vi "Close CAN Communication queues.vi"(8 "error in":errorcluster, 11 "CAN Session In":T1) -> (0 "error out":errorcluster)   [LabVIEW 2016]
uses:
  Typedefs/CAN Refnum.ctl
  Typedefs/CAN Session Pointer.ctl
  Typedefs/CAN Communication References.ctl
  Typedefs/kill process notifier array.ctl
  Typedefs/Write Queue.ctl
  Typedefs/FPGA CAN Frame Cluster.ctl
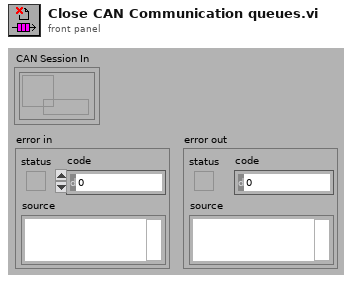
[diagram p1: front panel]
types:
  T1 = typedef "CAN Refnum.ctl" = refnum<k1>
  T2 = typedef "kill process notifier array.ctl" = refnum<notifier>[]
  T3 = typedef "Write Queue.ctl" = refnum<queue>
  T4 = typedef "CAN Session Pointer.ctl" = refnum<queue>
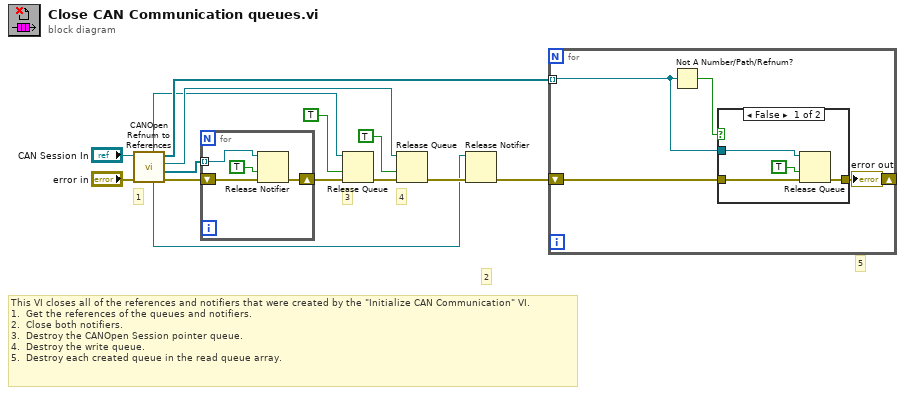
[diagram p0: block diagram]
diagram:
  # "This VI closes all of the references and notifiers that were created by the \"Initialize CAN Communication\" VI.\n1.  Get the references of the queues and notifiers.\n2.  Close both notifiers.\n3.  Destroy the CANOpen Session pointer queue.\n4.  Destroy the write queue.\n5.  Destroy each created queue in the read queue array."
  # "5"
  # "4"
  # "3"
  # "2"
  # "1"
  n1 = call "CANOpen Refnum to References.vi"("error in (no error)"="error in", "CAN Session In"="CAN Session In") -> ("error out"=w7:errorcluster, "kill process notifier array"=w5:T2, "Write Queue"=w13:T3, "Read Queue Array"=w11:T3[], "New Frame Notifier"=w1:refnum<notifier>, "CAN Session Queue"=w4:T4)  [unwired: 4 out]
  n2 = for {
    shift-right: [w18] -> w6
    shift-left: w7 -> [w19]
    tunnel: w5 -> [w16] mode=indexing
    n3 = Release Notifier(notifier=w16, force destroy? (F)=TRUE, error in (no error)=w19) -> (error out=w18:errorcluster)  [unwired: 2 out]
  }
  n4 = Release Queue(queue=w4, force destroy? (F)=TRUE, error in (no error)=w6) -> (error out=w9:errorcluster)  [unwired: 2 out]
  n5 = Release Queue(queue=w13, force destroy? (F)=TRUE, error in (no error)=w9) -> (error out=w3:errorcluster)  [unwired: 2 out]
  n6 = Release Notifier(notifier=w1, error in (no error)=w3) -> (error out=w2:errorcluster)  [unwired: 1 in, 2 out]
  n7 = for {
    tunnel: w11 -> [w20] mode=indexing
    shift-right: [w22] -> w8
    shift-left: w2 -> [w21]
    n8 = Not A Number/Path/Refnum?(number/path/refnum=w20) -> (NaN/Path/Refnum?=w23:bool)
    n9 = case shown="False" w23 {
      tunnel: w20 -> [w27 _]
      tunnel: [w26 w28] -> w22
      tunnel: w21 -> [w25 w28]
      frame False {
        n10 = Release Queue(queue=w27, force destroy? (F)=TRUE, error in (no error)=w25) -> (error out=w26:errorcluster)  [unwired: 2 out]
      }
      frame True {
      }
    }
  }
  "error out" <- w8
